vi "Concatenate PostPostMsg Message.vi"(9 "Source":string, 10 "Arguments":string, 11 "Async-Message":string) -> (3 "PostPostMsg Message":string)   [LabVIEW 2017, in "CSM Shared.lvlib"]
uses:
  CSM Shared.lvlib
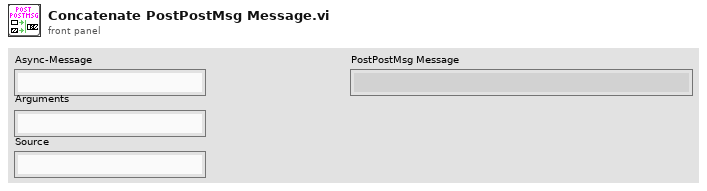
[diagram p1: front panel]
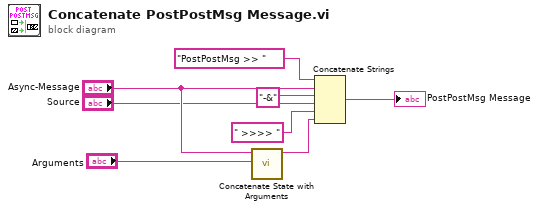
[diagram p0: block diagram]
diagram:
  n1 = call "Concatenate State with Arguments.vi"("Arguments"="Arguments", "State"="Async-Message") -> ("State With Arguements"=w1:string)  [unwired: 9 in]
  n2 = Concatenate Strings("PostPostMsg >> " ("State(s) at Back (\"\")"), "Async-Message", "-&" ("string"), "Source", " >>>> " ("string"), w1) -> (→"PostPostMsg Message":string)
